vi "is Result Ready.vi"(8 "error in (no error)":errorcluster, 11 "Cap Bank Interface in":refnum<class "Cap Bank Interface.lvclass">) -> (0 "error out":errorcluster, 2 "Result Available":bool=TRUE, 3 "Cap Bank Interface out":refnum<class "Cap Bank Interface.lvclass">)   [LabVIEW 2015, in "Cap Bank Interface.lvclass"]
uses:
  Cap Bank Interface.lvclass
  Cap Bank Interface.lvclass/Cap Bank Interface.ctl
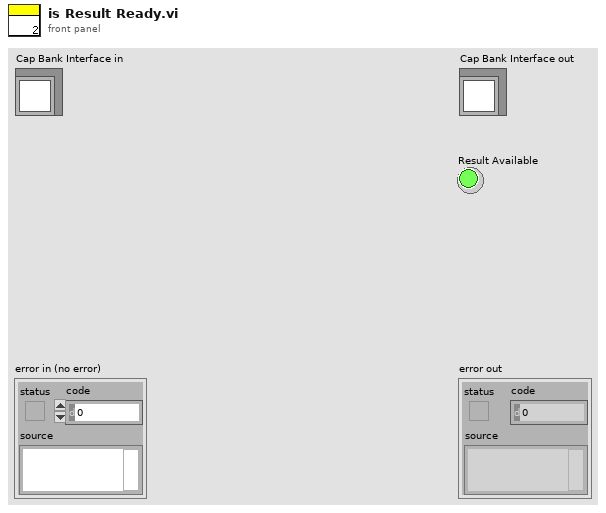
[diagram p1: front panel]
types:
  T1 = typedef "OPC connections.ctl" = cluster{"Data received":refnum<k13>, "Data Ready":refnum<k13>, "Message":refnum<k13>}
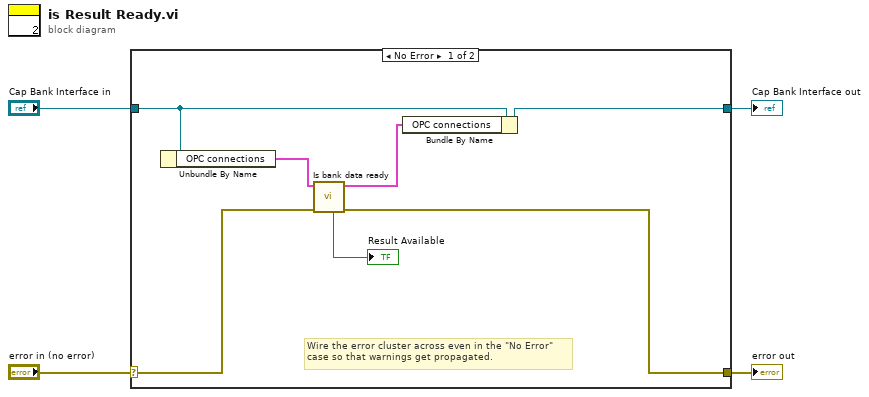
[diagram p0: block diagram]
diagram:
  n1 = case shown="No Error" "error in (no error)" {
    selector: "error in (no error)" -> [w7 w13]
    tunnel: [w6 w13] -> w3
    tunnel: [w9 w12] -> w1
    tunnel: "Cap Bank Interface in" -> [w11 w12]
    frame No Error {
      # "Wire the error cluster across even in the \"No Error\"\ncase so that warnings get propagated."
      n2 = Unbundle By Name(w11) -> ("OPC connections"=w10:T1)
      n3 = call "Is bank data ready.vi"("error IO"=w7, "OPC connections"=w10) -> ("error out"=w6:errorcluster, "OPC connections out"=w8:T1, "Data ready"=→"Result Available":bool)  [unwired: 7 in]
      n4 = Bundle By Name(cluster=w11, "OPC connections"=w8) -> (w9:refnum<class "Cap Bank Interface.lvclass">)
    }
    frame Error {
    }
  }
  "error out" <- w3
  "Cap Bank Interface out" <- w1
